vi "Sequencer Event Timeout--constant.vi"() -> (0 "Event Timeout (ms)":i32=100)   [LabVIEW 2024, in "Auto Modo.lvlib"]
uses:
  Auto Modo.lvlib
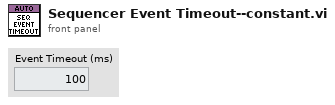
[diagram p1: front panel]
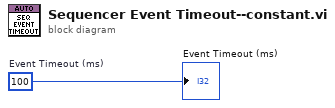
[diagram p0: block diagram]
diagram:
  w1 = 100  # Event Timeout (ms)
  "Event Timeout (ms)" <- w1
